vi "Int2Fxp.vi"(11 "Raw Voltage Input [Int.]":i64) -> (3 "Analog Volt Out [FXP.]":fxp<+/-,22,5>)   [LabVIEW 2018, in "FPGA functions.lvlib"]
doc: "Convert integer values to fixed point using 10 point moving average for easier multiplication."
uses:
  FPGA functions.lvlib
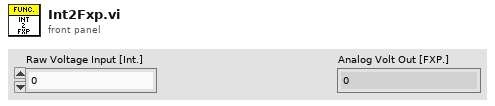
[diagram p1: front panel]
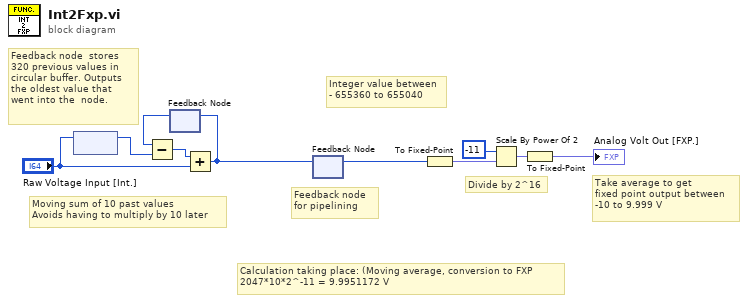
[diagram p0: block diagram]
diagram:
  # "Calculation taking place: (Moving average, conversion to FXP\n2047*10*2^-11 = 9.9951172 V"
  # "Feedback node  stores \n320 previous values in \ncircular buffer. Outputs \nthe oldest value that \nwent into the  node."
  # "Feedback node \nfor pipelining"
  # "Divide by 2^16"
  # "Integer value between\n- 655360 to 655040"
  # "Take average to get \nfixed point output between\n-10 to 9.999 V"
  # "Moving sum of 10 past values\nAvoids having to multiply by 10 later"
  n1 = feedback #1() -> (w8:i64)  [unwired: 1 in]
  n2 = feedback-in #1("Raw Voltage Input [Int.]") -> ()
  n3 = feedback #2() -> (w9:i64)  [unwired: 1 in]
  n4 = Subtract(x=w9, y=w8) -> (x-y=w10:i64)
  n5 = Add(x=w10, y="Raw Voltage Input [Int.]") -> (x+y=w1:i64)
  n6 = feedback-in #2(w1) -> ()
  n7 = feedback #3() -> (w3:i64)  [unwired: 1 in]
  n8 = feedback-in #3(w1) -> ()
  n9 = To Fixed-Point(number=w3) -> (fixed-point=w5:fxp<+/-,38,21>)  [unwired: 1 out]
  n10 = Scale By Power Of 2(n=-11, x=w5) -> (x*2^n=w4:fxp<+/-,38,21>)
  n11 = To Fixed-Point(number=w4) -> (fixed-point=→"Analog Volt Out [FXP.]":fxp<+/-,22,5>)  [unwired: 1 out]
